vi "Fur_Limit.vi"(9 "Furnace Temp":dbl, 10 "Eurotherm Input":dbl, 11 "Fur Limit":dbl) -> (2 "Signal Out":dbl(knob) scale=0.0..10.0)   [LabVIEW 2014]
panel:
  # "Furnace Limit Vi"
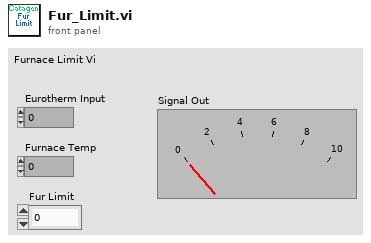
[diagram p1: front panel]
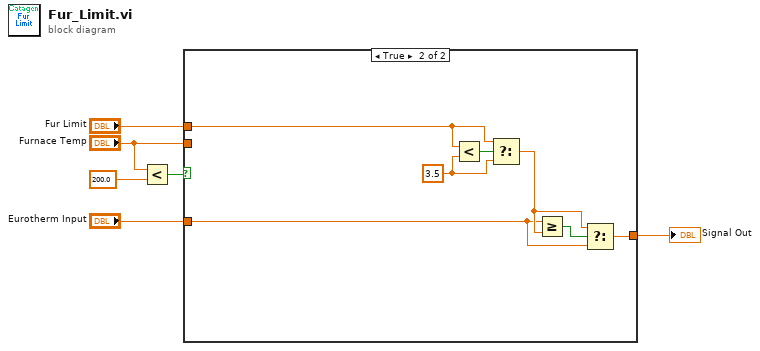
[diagram p0: block diagram]
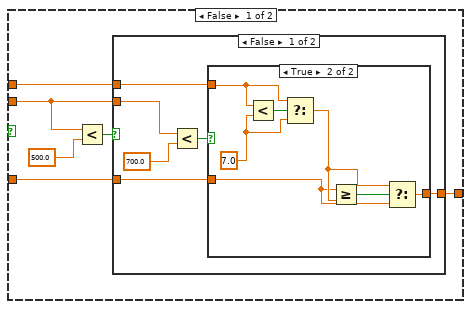
[diagram p2: hidden frame]
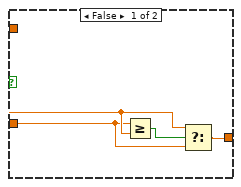
[diagram p3: hidden frame]
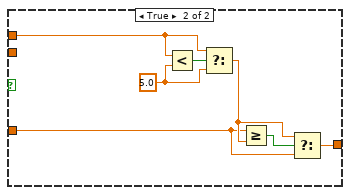
[diagram p4: hidden frame]
diagram:
  n1 = Less?(x="Furnace Temp", y=200.0) -> (x < y?=w5:bool)
  n2 = case shown="True" w5 {
    tunnel: "Furnace Temp" -> [w8 _]
    tunnel: [w9 w40] -> w1
    tunnel: "Eurotherm Input" -> [w10 w38]
    tunnel: "Fur Limit" -> [w7 w42]
    frame False {
      n3 = Less?(x=w8, y=500.0) -> (x < y?=w11:bool)
      n4 = case shown="False" w11 {
        tunnel: w10 -> [w14 w32]
        tunnel: [w15 w30] -> w9
        tunnel: w8 -> [w17 _]
        tunnel: w7 -> [w13 w34]
        frame False {
          n5 = Less?(x=w17, y=700.0) -> (x < y?=w16:bool)
          n6 = case shown="True" w16 {
            tunnel: [w22 w23] -> w15
            tunnel: w14 -> [w20 w25]
            tunnel: w13 -> [w21 w28]
            frame False {
              n7 = Greater Or Equal?(x=w20, y=w21) -> (x >= y?=w19:bool)
              n8 = Select(t=w21, s=w19, f=w20) -> (s? t:f=w22:dbl)
            }
            frame True {
              w27 = 7.0 ("y")
              n9 = Less?(x=w28, y=w27) -> (x < y?=w29:bool)
              n10 = Select(t=w28, s=w29, f=w27) -> (s? t:f=w26:dbl)
              n11 = Greater Or Equal?(x=w25, y=w26) -> (x >= y?=w24:bool)
              n12 = Select(t=w26, s=w24, f=w25) -> (s? t:f=w23:dbl)
            }
          }
        }
        frame True {
          w36 = 5.0 ("Fur Limit")
          n13 = Less?(x=w34, y=w36) -> (x < y?=w35:bool)
          n14 = Select(t=w34, s=w35, f=w36) -> (s? t:f=w33:dbl)
          n15 = Greater Or Equal?(x=w32, y=w33) -> (x >= y?=w31:bool)
          n16 = Select(t=w33, s=w31, f=w32) -> (s? t:f=w30:dbl)
        }
      }
    }
    frame True {
      w41 = 3.5 ("Fur Limit")
      n17 = Less?(x=w42, y=w41) -> (x < y?=w43:bool)
      n18 = Select(t=w42, s=w43, f=w41) -> (s? t:f=w39:dbl)
      n19 = Greater Or Equal?(x=w38, y=w39) -> (x >= y?=w37:bool)
      n20 = Select(t=w39, s=w37, f=w38) -> (s? t:f=w40:dbl)
    }
  }
  "Signal Out" <- w1
